vi "Editor UI Initialze.vi"(8 "error in (no error)":errorcluster, 11 "Editor.lvclass in":refnum<data-value>) -> (0 "error out":errorcluster, 3 "Editor.lvclass out":refnum<data-value>)   [LabVIEW 2015, in "Editor.lvclass"]
uses:
  Editor.lvclass
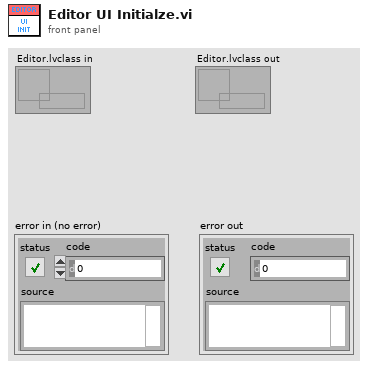
[diagram p1: front panel]
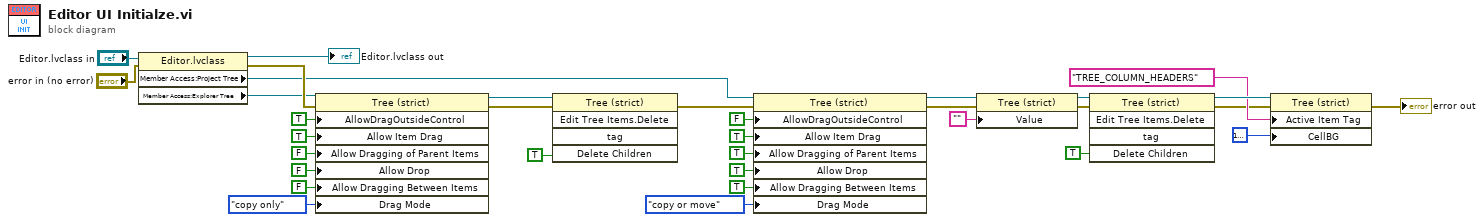
[diagram p0: block diagram]
diagram:
  n1 = property class="Editor.lvclass"(reference="Editor.lvclass in", error in="error in (no error)") -> (reference out=→"Editor.lvclass out":refnum<data-value>, error out=w9:errorcluster, "Member Access:Project Tree"=w7:refnum<vi>, "Member Access:Explorer Tree"=w8:refnum<vi>)
  n2 = property class="Tree (strict)"(reference=w8, error in=w9, "AllowDragOutsideControl"=TRUE ("Drag/Drop:Allow Drag and Drop Outside Control"), "Allow Item Drag"=TRUE ("Drag/Drop:Allow Dragging"), "Allow Dragging of Parent Items"=FALSE ("Drag/Drop:Allow Dragging of Parent Items"), "Allow Drop"=FALSE ("Drag/Drop:Allow Dropping"), "Allow Dragging Between Items"=FALSE ("Drag/Drop:Allow Dropping Between Items"), "Drag Mode"=enum32{"copy or move", "copy only", "move only"}."copy only" ("Drag/Drop:Drag Mode")) -> (reference out=w28:refnum<vi>, error out=w27:errorcluster)
  n3 = invoke class="Tree (strict)" method="Edit Tree Items.Delete"(reference=w28, error in=w27, "Delete Children"=TRUE) -> (error out=w14:errorcluster)  [unwired: 2 in, 4 out]
  n4 = property class="Tree (strict)"(reference=w7, error in=w14, "AllowDragOutsideControl"=FALSE ("Drag/Drop:Allow Drag and Drop Outside Control"), "Allow Item Drag"=TRUE ("Drag/Drop:Allow Dragging"), "Allow Dragging of Parent Items"=TRUE ("Drag/Drop:Allow Dragging of Parent Items"), "Allow Drop"=TRUE ("Drag/Drop:Allow Dropping"), "Allow Dragging Between Items"=TRUE ("Drag/Drop:Allow Dropping Between Items"), "Drag Mode"=enum32{"copy or move", "copy only", "move only"}."copy or move" ("Drag/Drop:Drag Mode")) -> (reference out=w13:refnum<vi>, error out=w12:errorcluster)
  n5 = property class="Tree (strict)"(reference=w13, error in=w12, "Value"="") -> (reference out=w30:refnum<vi>, error out=w31:errorcluster)
  n6 = invoke class="Tree (strict)" method="Edit Tree Items.Delete"(reference=w30, error in=w31, "Delete Children"=TRUE ("Delete Children?")) -> (reference out=w5:refnum<vi>, error out=w3:errorcluster)  [unwired: 2 in, 3 out]
  n7 = property class="Tree (strict)"(reference=w5, error in=w3, "Active Item Tag"="TREE_COLUMN_HEADERS", "CellBG"=u32 16777238) -> (error out=→"error out":errorcluster)  [unwired: 1 out]
